vi "number1_global.vi"() -> ()   [LabVIEW 2014]
panel:
  out "Acquire Data button":bool
  out "config ok button":bool
  in  "#s":dbl
  in  "Fs":dbl
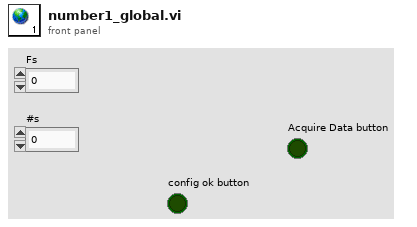
[diagram p1: front panel]
diagram:
